vi "Configure Frequency Ratio.vi"(8 "error in (no error)":errorcluster, 9 "Frequency Ratio Estimate (1)":dbl=1.0, 10 "Frequency Ratio (0:Input 1:2)":i32(ring) items=["Input 1:2", "Input 1:3", "Input 2:1", "Input 3:1"], 11 "VISA resource name":refnum<visa-resource-name>) -> (0 "error out":errorcluster, 3 "VISA resource name out":refnum<visa-resource-name>)   [LabVIEW 2013, in "Counter.lvlib" / "PICOTEST U62XXA series.lvlib"]
doc: "Configures settings required for a Frequency Ratio Measurement.\n\n<B>Note:</B>\nThe U6220A <B>does not</B> support the \"Frequency Ratio\" commands.\n\nThe measurement arming is coupled to Digits. Arming can be changed by calling any of the Arming VIs. The measurement channel has auto-trigger enabled at 50% with a positive slope."
uses:
  PICOTEST U62XXA series.lvlib
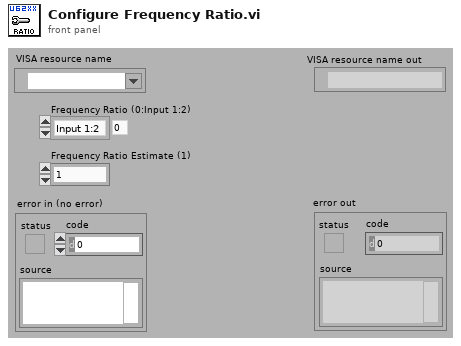
[diagram p1: front panel]
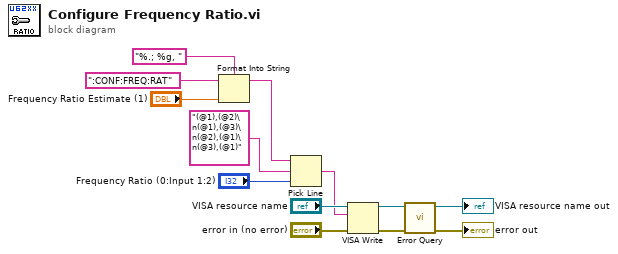
[diagram p0: block diagram]
diagram:
  n1 = Format Into String(format string="%.; %g, ", initial string=":CONF:FREQ:RAT" ("string (\"\")"), "Frequency Ratio Estimate (1)") -> (resulting string=w5:string)  [unwired: 1 in, 1 out]
  n2 = Pick Line(string ("")=w5, multi-line string="(@1),(@2)\n(@1),(@3)\n(@2),(@1)\n(@3),(@1)", line index="Frequency Ratio (0:Input 1:2)") -> (output string=w9:string)
  n3 = VISA Write(VISA resource name="VISA resource name", write buffer=w9, error in (no error)="error in (no error)") -> (VISA resource name out=w4:refnum<visa-resource-name>, error out=w2:errorcluster)  [unwired: 1 out]
  n4 = call "Error Query.vi"("error in (no error)"=w2, "VISA resource name"=w4) -> ("error out"=→"error out":errorcluster, "VISA resource name out"=→"VISA resource name out":refnum<visa-resource-name>)  [unwired: 6 in, 2 out]
